vi "Copy Limits File.vi"(8 "error in (no error)":errorcluster, 11 "Limits File Path In":path) -> (0 "error out":errorcluster, 3 "Limits File Path Out":path)   [LabVIEW 2018, in "niRFSTS Sequence Flow.lvclass"]
uses:
  niRFSTS Sequence Flow.lvclass
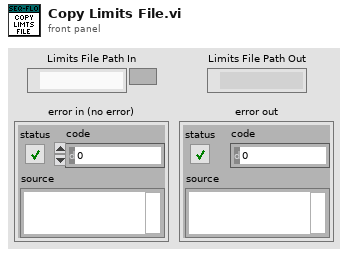
[diagram p1: front panel]
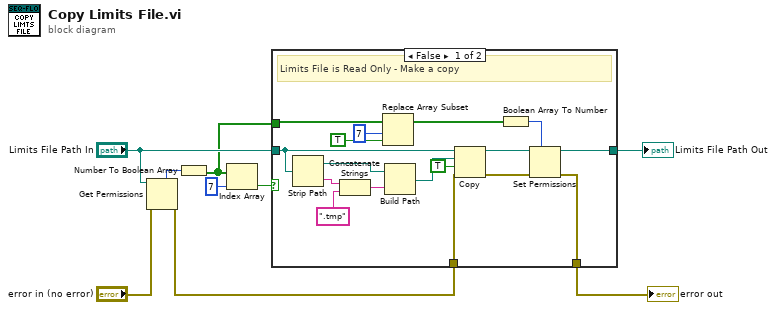
[diagram p0: block diagram]
diagram:
  n1 = Get Permissions(8:"error in (no error)", 11:"Limits File Path In") -> (0:w2:errorcluster, 5:w8:i16)  [unwired: 3 out]
  n2 = Number To Boolean Array(number=w8) -> (Boolean array=w1:bool[])
  n3 = Index Array(array=w1, index=7) -> (element=w6:bool)
  n4 = case shown="False" w6 {
    tunnel: "Limits File Path In" -> [w26 w28]
    tunnel: [w17 w28] -> w4
    tunnel: [w15 w27] -> w3
    tunnel: w2 -> [w22 w27]
    tunnel: w1 -> [w14 _]
    frame False {
      # "Limits File is Read Only - Make a copy"
      n5 = Strip Path(path=w26) -> (stripped path=w21:path, name=w19:string)
      n6 = Concatenate Strings(w19, ".tmp" ("name or relative path")) -> (w20:string)
      n7 = Replace Array Subset(array=w14, new element=TRUE ("new element/subarray"), index=7) -> (w11:bool[])
      n8 = Build Path(base path=w21, name or relative path=w20) -> (appended path=w24:path)
      n9 = Copy(8:w22, 9:TRUE ("overwrite (F)"), 10:w24, 11:w26) -> (0:w16:errorcluster, 3:w18:path)  [unwired: 1 in, 1 out]
      n10 = Boolean Array To Number(Boolean array=w11) -> (number=w10:u32)
      n11 = Set Permissions(7:w10, 8:w16, 11:w18) -> (0:w15:errorcluster, 3:w17:path)  [unwired: 2 in]
    }
    frame True {
      # "Limits file writeable make changes directly"
    }
  }
  "error out" <- w3
  "Limits File Path Out" <- w4
